vi "Report.vi"(1 "Message":string, 2 "current vi path":path) -> ()   [LabVIEW 2011]
uses:
  GlobalPath.vi
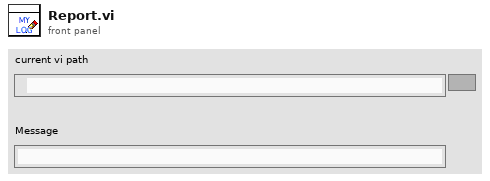
[diagram p1: front panel]
types:
  T1 = enum16{"open", "replace", "create", "open or create", "replace or create", "replace or create with confirmation"}
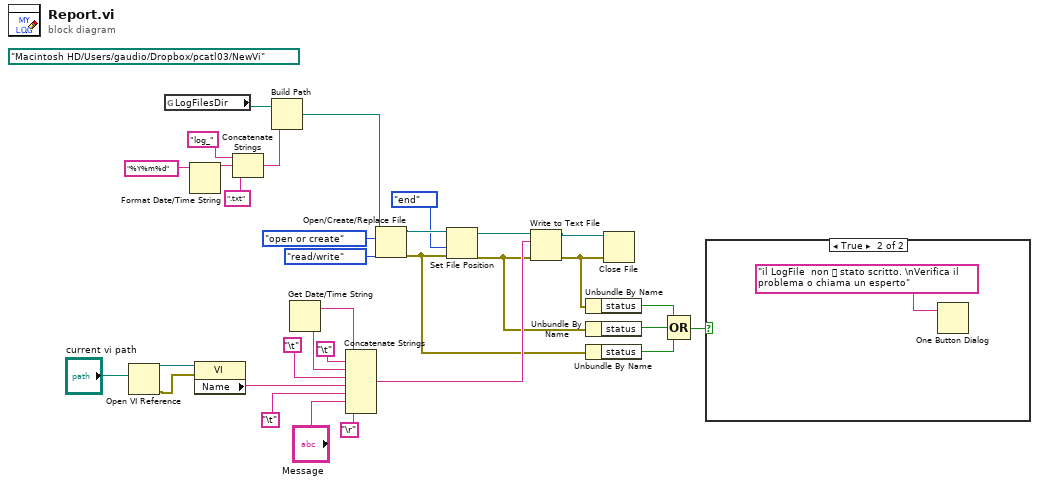
[diagram p0: block diagram]
diagram:
  (unwired) path "/Macintosh HD/Users/gaudio/Dropbox/pcatl03/NewVi" ("base path")
  n1 = Open VI Reference(vi path="current vi path") -> (vi reference=w16:refnum<vi>, error out=w15:errorcluster)  [unwired: 5 in]
  n2 = global read "GlobalPath.vi" "LogFilesDir"() -> (w1:path)
  n3 = Format Date/Time String(time format string (%c)="%Y%m%d") -> (date/time string=w20:string)  [unwired: 2 in]
  n4 = property class="VI"(reference=w16, error in=w15) -> ("Name"=w9:string)  [unwired: 2 out]
  n5 = Concatenate Strings("log_" ("string"), w20, ".txt" ("string")) -> (w18:string)
  n6 = Build Path(base path=w1, name or relative path=w18) -> (appended path=w17:path)
  n7 = Get Date/Time String() -> (date string=w25:string, time string=w24:string)  [unwired: 3 in]
  n8 = Concatenate Strings(w25, "\t", w24, "\t", w9, "\t", "Message", "\r") -> (w27:string)
  n9 = Open/Create/Replace File(file path (use dialog)=w17, operation (0:open)=T1."open or create", access (0:read/write)=enum16{"read/write", "read-only", "write-only"}."read/write") -> (refnum out=w29:refnum<file>, error out=w7:errorcluster)  [unwired: 3 in, 1 out]
  n10 = Set File Position(refnum=w29, from (0:start)=enum16{"start", "end", "current"}."end", error in=w7) -> (refnum out=w28:refnum<file>, error out=w6:errorcluster)  [unwired: 1 in]
  n11 = Write to Text File(file (use dialog)=w28, text=w27, error in=w6) -> (refnum out=w31:refnum<file>, error out=w8:errorcluster)  [unwired: 1 in, 1 out]
  n12 = Unbundle By Name(w8) -> ("status"=w5:bool)
  n13 = Unbundle By Name(w6) -> ("status"=w4:bool)
  n14 = Unbundle By Name(w7) -> ("status"=w3:bool)
  n15 = Close File(refnum=w31, error in=w8) -> ()  [unwired: 2 out]
  n16 = Compound Arithmetic op=OR(w5, w4, w3) -> (w2:bool)
  n17 = case shown="True" w2 {
    frame False {
    }
    frame True {
      n18 = One Button Dialog(message="il LogFile  non  stato scritto. \nVerifica il problema o chiama un esperto") -> ()  [unwired: 1 in, 1 out]
    }
  }
